vi "NO_____Auto_Routine_LeftTwoPiece.vi"   [LabVIEW 2023]
uses:
  Arm2/ArmGetSetpointEnum.ctl
types:
  T1 = typedef "ArmGetSetpointEnum.ctl" = enum16{"ArmFloorPickup", "ArmAmpDeposit", "ArmSpeakerShoot", "ArmStartPosition", "ArmRestPosition", "ArmSourceIntake", "ArmAwayShoot"}
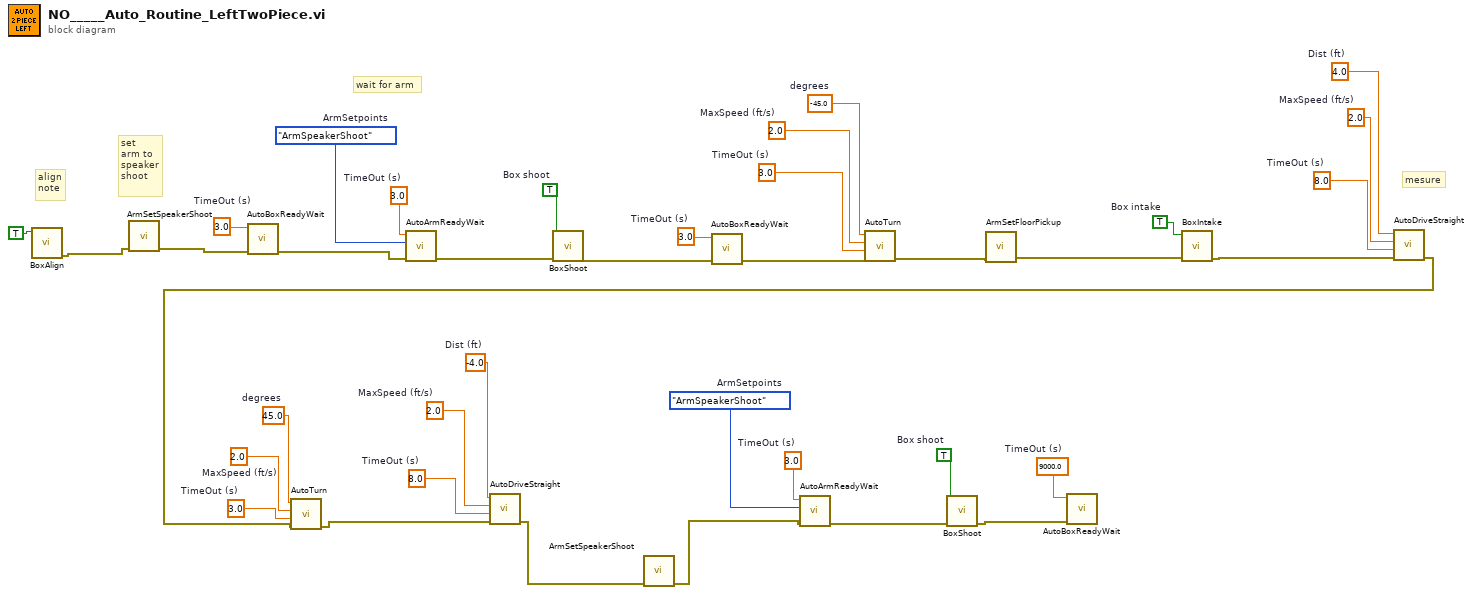
[diagram p0: block diagram]
diagram:
  w3 = 3.0  # TimeOut (s)
  w35 = 8.0  # TimeOut (s)
  w34 = 2.0  # MaxSpeed (ft/s)
  w33 = -4.0  # Dist (ft)
  w32 = 8.0  # TimeOut (s)
  w31 = 2.0  # MaxSpeed (ft/s)
  w30 = 4.0  # Dist (ft)
  w28 = 9000.0  # TimeOut (s)
  w27 = 3.0  # TimeOut (s)
  w26 = 2.0  # MaxSpeed (ft/s)
  w25 = 45.0  # degrees
  w24 = TRUE  # Box shoot
  w23 = ArmGetSetpointEnum."ArmSpeakerShoot"  # ArmSetpoints
  w22 = 3.0  # TimeOut (s)
  w19 = 3.0  # TimeOut (s)
  w18 = 2.0  # MaxSpeed (ft/s)
  w17 = -45.0  # degrees
  w14 = TRUE  # Box intake
  w13 = TRUE  # Box shoot
  w12 = ArmGetSetpointEnum."ArmSpeakerShoot"  # ArmSetpoints
  w11 = 3.0  # TimeOut (s)
  w6 = 3.0  # TimeOut (s)
  # "set \narm to\nspeaker\nshoot"
  # "align\nnote"
  # "mesure"
  # "wait for arm"
  n1 = call "BoxAlign.vi"("box align"=TRUE) -> ("error out"=w4:errorcluster)  [unwired: 10 in]
  n2 = call "ArmSetSpeakerShoot.vi"("error in (no error)"=w4) -> ("error out"=w2:errorcluster)  [unwired: 10 in]
  n3 = call "AutoBoxReadyWait.vi"("error in (no error)"=w2, "TimeOut (s)"=w3) -> ("error out"=w1:errorcluster)  [unwired: 9 in]
  n4 = call "AutoArmReadyWait.vi"("error in (no error)"=w1, "ArmSetpoints"=w12, "TimeOut (s)"=w11) -> ("error out"=w7:errorcluster)  [unwired: 8 in]
  n5 = call "BoxShoot.vi"("error in (no error)"=w7, "Box shoot"=w13) -> ("error out"=w8:errorcluster)  [unwired: 9 in]
  n6 = call "AutoBoxReadyWait.vi"("error in (no error)"=w8, "TimeOut (s)"=w6) -> ("error out"=w15:errorcluster)  [unwired: 9 in]
  n7 = call "AutoTurn.vi"("error in (no error)"=w15, "TimeOut (s)"=w19, "MaxSpeed (ft/s)"=w18, "degrees"=w17) -> ("error out"=w16:errorcluster)  [unwired: 7 in]
  n8 = call "ArmSetFloorPickup.vi"("error in (no error)"=w16) -> ("error out"=w9:errorcluster)  [unwired: 10 in]
  n9 = call "BoxIntake.vi"("error in (no error)"=w9, "Box intake"=w14) -> ("error out"=w10:errorcluster)  [unwired: 9 in]
  n10 = call "AutoDriveStraight.vi"("error in (no error)"=w10, "TimeOut (s)"=w32, "MaxSpeed (ft/s)"=w31, "Dist (ft)"=w30) -> ("error out"=w38:errorcluster)  [unwired: 7 in]
  n11 = call "AutoTurn.vi"("error in (no error)"=w38, "TimeOut (s)"=w27, "MaxSpeed (ft/s)"=w26, "degrees"=w25) -> ("error out"=w37:errorcluster)  [unwired: 7 in]
  n12 = call "AutoDriveStraight.vi"("error in (no error)"=w37, "TimeOut (s)"=w35, "MaxSpeed (ft/s)"=w34, "Dist (ft)"=w33) -> ("error out"=w36:errorcluster)  [unwired: 7 in]
  n13 = call "ArmSetSpeakerShoot.vi"("error in (no error)"=w36) -> ("error out"=w20:errorcluster)  [unwired: 10 in]
  n14 = call "AutoArmReadyWait.vi"("error in (no error)"=w20, "ArmSetpoints"=w23, "TimeOut (s)"=w22) -> ("error out"=w21:errorcluster)  [unwired: 8 in]
  n15 = call "BoxShoot.vi"("error in (no error)"=w21, "Box shoot"=w24) -> ("error out"=w29:errorcluster)  [unwired: 9 in]
  n16 = call "AutoBoxReadyWait.vi"("error in (no error)"=w29, "TimeOut (s)"=w28) -> ()  [unwired: 9 in, 1 out]
